vi "RotationMartix.vi"   [LabVIEW 2014]
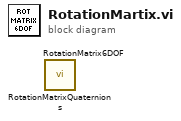
[diagram p0: block diagram]
diagram:
  n1 = call "RotationMatrixQuaternions.vi"() -> ()  [unwired: 1 in, 1 out]
  n2 = call "RotationMatrix6DOF.vi"() -> ()  [unwired: 1 in, 1 out]
